vi "Set Defer Updates.vi"(8 "error in (no error)":errorcluster, 10 "Defer Updates":bool, 11 "2DArrayManager in":refnum<class "2DArrayManager.lvclass">) -> (0 "error out":errorcluster, 3 "2DArrayManager out":refnum<class "2DArrayManager.lvclass">)   [LabVIEW 2020, in "OOPanel.lvlib" / "2DArrayManager.lvclass"]
uses:
  2DArrayManager.lvclass
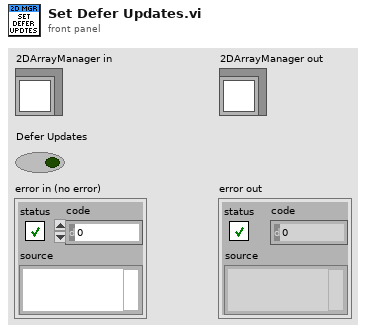
[diagram p1: front panel]
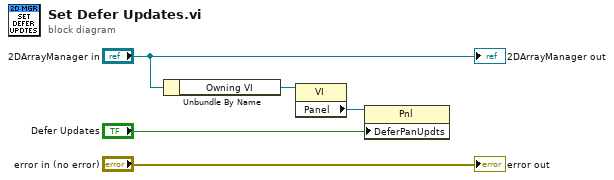
[diagram p0: block diagram]
diagram:
  n1 = Unbundle By Name("2DArrayManager in") -> ("Owning VI"=w2:refnum<vi>)
  n2 = property class="VI"(reference=w2) -> ("Panel"=w1:refnum<vi>)  [unwired: 1 in, 2 out]
  n3 = property class="Pnl"(reference=w1, "DeferPanUpdts"="Defer Updates") -> ()  [unwired: 1 in, 2 out]
  "error out" <- "error in (no error)"
  "2DArrayManager out" <- "2DArrayManager in"
